vi "Weather Station UI.vi"() -> ()   [LabVIEW 2022 SP3]
doc: "This is the main VI in the Weather Station project. It contains the user interface for a temperature warning system. Temperature is retrieved every half second; data is logged when a warning has occurred."
uses:
  Weather Station States.ctl
  Supporting Files/Weather Data.ctl
  Instance           2 26Saved   Weather Station UI .vi
panel:
  out "Warning":string
  in  "Lower Limit":dbl=20.0
  in  "Upper Limit":dbl=30.0
  in  "Stop Button":bool
  out "Temperature History":dbl(graph)
  # "Temperature Ranges (C)"
  # "Freeze"
  # "Heat \nStroke"
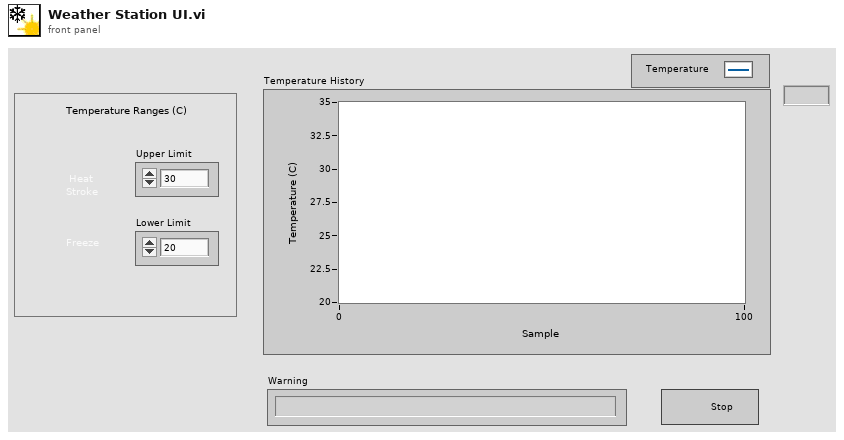
[diagram p1: front panel]
types:
  T1 = typedef "Weather Data.ctl" = cluster{"Current Temperature":dbl, "Max Temperature":dbl, "Min Temperature":dbl, "Temperature Warning?":bool, "Temperature Warning Text":string}
  T2 = typedef "Weather Station States.ctl" = enum16{"Acquisition", "Analysis", "Data Log", "Time Check"}
  T3 = enum16{"open", "replace", "create", "open or create", "replace or create", "replace or create with confirmation"}
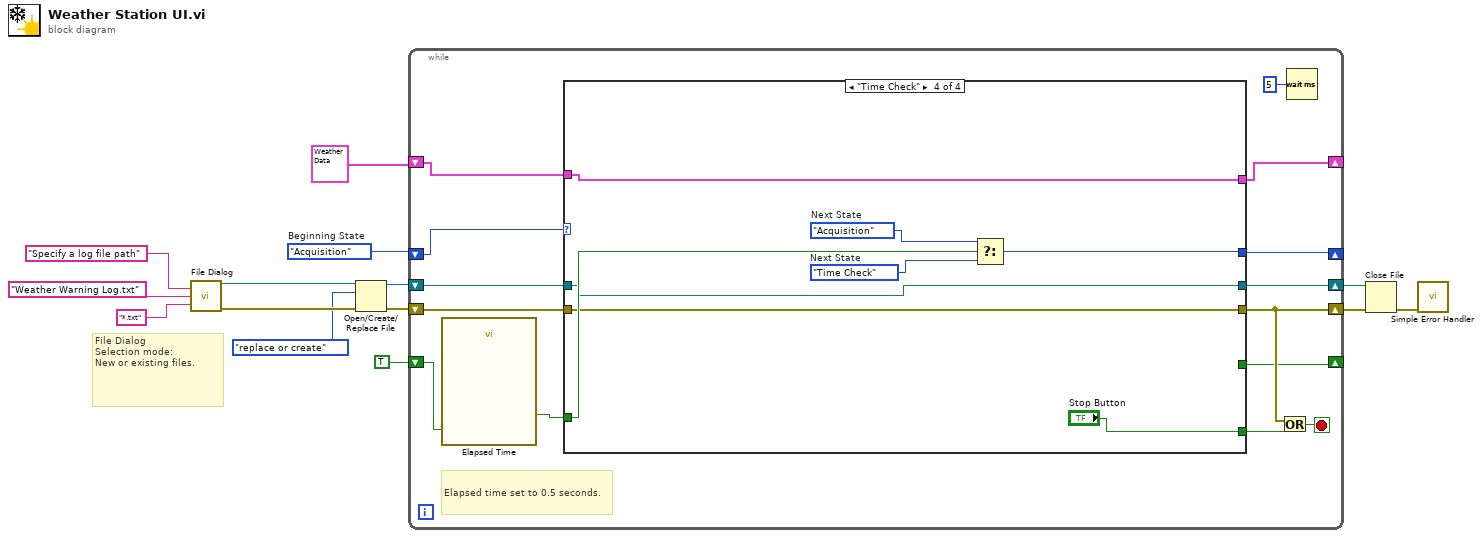
[diagram p0: block diagram]
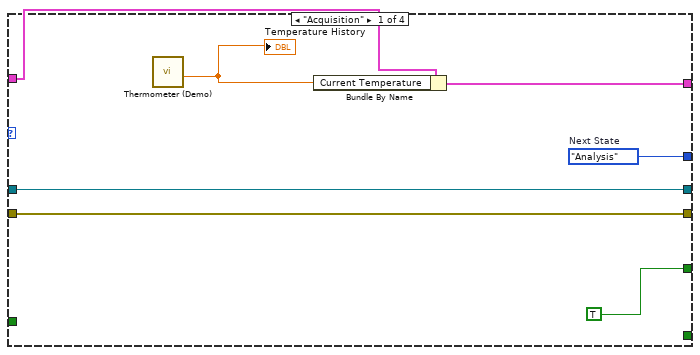
[diagram p2: hidden frame]
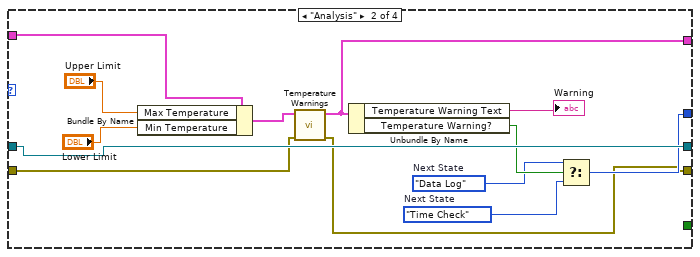
[diagram p3: hidden frame]
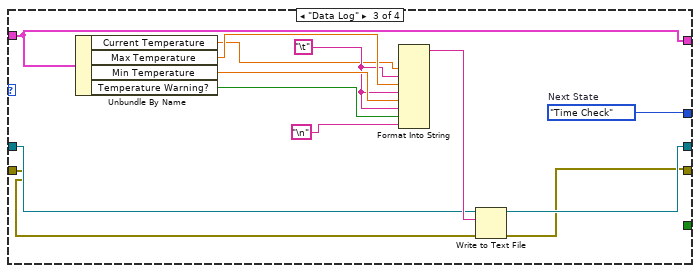
[diagram p4: hidden frame]
diagram:
  w2 = Weather_Station_States."Acquisition"  # Beginning State
  # "File Dialog\nSelection mode:\nNew or existing files."
  n1 = call "File Dialog"("prompt"="Specify a log file path", "default name"="Weather Warning Log.txt", "pattern (all files)"="*.txt" ("pattern label")) -> ("selected path"=w8:path, "error out"=w5:errorcluster)  [unwired: 9 in, 2 out]
  n2 = Open/Create/Replace File(file path (use dialog)=w8, error in=w5, operation (0:open)=T3."replace or create") -> (refnum out=w10:refnum<file>, error out=w9:errorcluster)  [unwired: 3 in, 1 out]
  n3 = while {
    shift-right: [w21] -> w14
    shift-left: w9 -> [w28]
    shift-right: [w26] -> w13
    shift-left: w10 -> [w25]
    shift-right: [w15] -> _
    shift-left: TRUE ("stop") -> [w23]
    shift-right: [w17] -> _
    shift-left: w2 -> [w20]
    shift-right: [w18] -> _
    shift-left: T1 {"Current Temperature"=0.0, "Max Temperature"=0.0, "Min Temperature"=0.0, "Temperature Warning?"=FALSE, "Temperature Warning Text"="No Warning"} ("Weather Data In") -> [w19]
    stop <- w27 stop-if-true
    # "Elapsed time set to 0.5 seconds."
    n4 = call "Elapsed Time"("Reset"=w23) -> ("Time has Elapsed"=w22:bool)  [unwired: 11 in, 7 out]
    n5 = case shown="\"Time Check\"" w20 {
      tunnel: [w34 w37 w50 w64] -> w21
      tunnel: w28 -> [w34 w44 w51 w64]
      tunnel: [w35 w45 w52 w65] -> w26
      tunnel: w25 -> [w35 w45 w53 w65]
      tunnel: w22 -> [_ _ _ w66]
      tunnel: w19 -> [w33 w48 w61 w69]
      tunnel: [w32 w42 w61 w69] -> w18
      tunnel: [w31 w38 w49 w63] -> w17
      tunnel: [TRUE _ _ _] -> w15
      tunnel: [_ _ _ "Stop Button"] -> w16
      frame "Acquisition" {
        w31 = Weather_Station_States."Analysis"  # Next State
        n6 = call "Thermometer (Demo).vi"() -> ("Temperature Value"=w29:dbl)  [unwired: 11 in]
        "Temperature History" <- w29
        n7 = Bundle By Name(cluster=w33, "Current Temperature"=w29) -> (w32:T1)
      }
      frame "Analysis" {
        w39 = Weather_Station_States."Time Check"  # Next State
        w40 = Weather_Station_States."Data Log"  # Next State
        n8 = Bundle By Name(cluster=w48, "Max Temperature"="Upper Limit", "Min Temperature"="Lower Limit") -> (w43:T1)
        n9 = call "Temperature Warnings.vi"("Error In"=w44, "Weather Data In"=w43) -> ("Error Out"=w37:errorcluster, "Weather Data Out"=w42:T1)  [unwired: 8 in]
        n10 = Unbundle By Name(w42) -> ("Temperature Warning Text"=→"Warning":string, "Temperature Warning?"=w41:bool)
        n11 = Select(t=w40, s=w41, f=w39) -> (s? t:f=w38:T2)
      }
      frame "Data Log" {
        w49 = Weather_Station_States."Time Check"  # Next State
        w56 = "\t"
        n12 = Unbundle By Name(w61) -> ("Current Temperature"=w55:dbl, "Max Temperature"=w57:dbl, "Min Temperature"=w58:dbl, "Temperature Warning?"=w60:bool)
        n13 = Format Into String(w55, w56, w57, w56, w58, w56, w60, "\n") -> (resulting string=w54:string)  [unwired: 3 in, 1 out]
        n14 = Write to Text File(file (use dialog)=w53, text=w54, error in=w51) -> (refnum out=w52:refnum<file>, error out=w50:errorcluster)  [unwired: 1 in, 1 out]
      }
      frame "Time Check" {
        w67 = Weather_Station_States."Time Check"  # Next State
        w68 = Weather_Station_States."Acquisition"  # Next State
        n15 = Select(t=w68, s=w66, f=w67) -> (s? t:f=w63:T2)
      }
    }
    n16 = Or(x=w21, y=w16) -> (x .or. y?=w27:bool)
    n17 = Wait (ms)(milliseconds to wait=u32 5 ("y")) -> ()  [unwired: 1 out]
  }
  n18 = Close File(refnum=w13, error in=w14) -> (error out=w12:errorcluster)  [unwired: 1 out]
  n19 = call <vilib>:"Simple Error Handler.vi"("error in (no error)"=w12) -> ()  [unwired: 4 in, 5 out]
